vi "Create Virtual Folder.vi"(10 "Folder Config":T1, 11 "Library":refnum<vi>) -> (3 "Folder Ref":refnum<vi>)   [LabVIEW 2020, in "Negentropic IDE.lvlib"]
uses:
  Negentropic IDE.lvlib
  Folder Config.ctl
  Scope.ctl
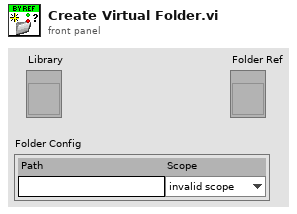
[diagram p1: front panel]
types:
  T1 = typedef "Negentropic IDE.lvlib/Folder Config.ctl" = cluster{"Path":string, "Scope":T2}
  T2 = typedef "Negentropic IDE.lvlib/Scope.ctl" = enum32{"invalid scope", "public", "private", "protected", "community"}
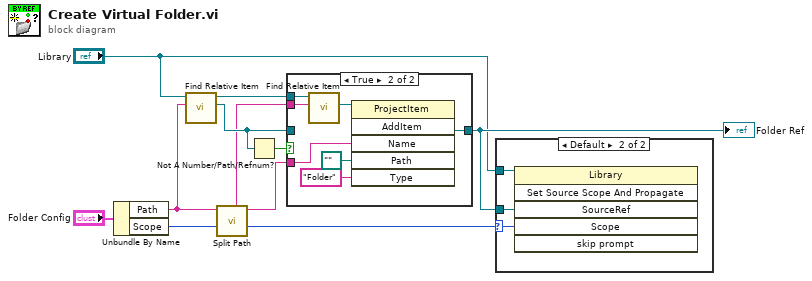
[diagram p0: block diagram]
diagram:
  n1 = Unbundle By Name("Folder Config") -> ("Path"=w5:string, "Scope"=w9:T2)
  n2 = call "Find Relative Item.vi"("Item Path"=w5, "Root Item In"="Library") -> ("Item Ref"=w3:refnum<vi>, "Root Item"=w1:refnum<vi>)  [unwired: 7 in, 1 out]
  n3 = call "Split Path.vi"("Item Path"=w5) -> ("Item Name"=w7:string, "Parent Path"=w2:string)  [unwired: 9 in]
  n4 = Not A Number/Path/Refnum?(number/path/refnum=w3) -> (NaN/Path/Refnum?=w4:bool)
  n5 = case shown="True" w4 {
    tunnel: w7 -> [_ w18]
    tunnel: [w11 w17] -> w8
    tunnel: w3 -> [w11 _]
    tunnel: w2 -> [_ w14]
    tunnel: w1 -> [_ w13]
    frame False {
    }
    frame True {
      n6 = call "Find Relative Item.vi"("Item Path"=w14, "Root Item In"=w13) -> ("Item Ref"=w12:refnum<vi>)  [unwired: 7 in, 2 out]
      n7 = invoke class="ProjectItem" method="AddItem"(reference=w12, "Name"=w18, "Path"=path "", "Type"="Folder") -> ("AddItem"=w17:refnum<vi>)  [unwired: 2 in, 5 out]
    }
  }
  "Folder Ref" <- w8
  n8 = case shown="Default" w9 {
    selector: w9 -> [_ w20]
    tunnel: "Library" -> [_ w21]
    tunnel: w8 -> [_ w19]
    frame "invalid scope" {
    }
    frame Default {
      n9 = invoke class="Library" method="Set Source Scope And Propagate"(reference=w21, "SourceRef"=w19, "Scope"=w20) -> ()  [unwired: 3 in, 6 out]
    }
  }
